vi "MotorMpas.vi"(2 "entrée d'erreur 2":errorcluster caption="entrée d'erreur", 3 "Parameter":i32) -> (0 "entrée d'erreur":errorcluster, 1 "Numérique":i32)   [LabVIEW 2009]
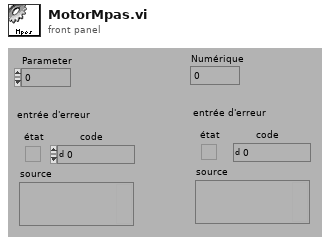
[diagram p1: front panel]
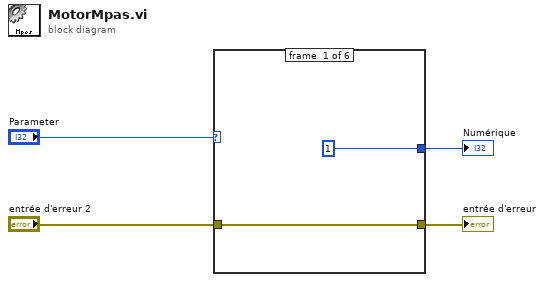
[diagram p0: block diagram]
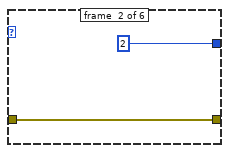
[diagram p2: hidden frame]
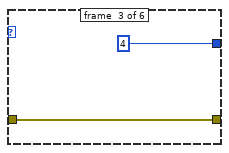
[diagram p3: hidden frame]
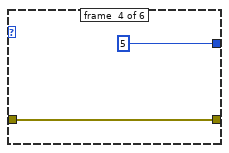
[diagram p4: hidden frame]
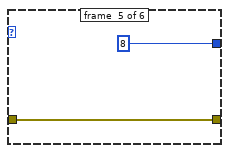
[diagram p5: hidden frame]
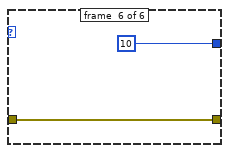
[diagram p6: hidden frame]
diagram:
  n1 = case shown="1, Default" "Parameter" {
    tunnel: "entrée d'erreur 2" -> [w6 w8 w10 w12 w14 w16]
    tunnel: [w6 w8 w10 w12 w14 w16] -> w4
    tunnel: [1 2 4 5 8 10] -> w3
    frame #0 {
    }
    frame #1 {
    }
    frame #2 {
    }
    frame #3 {
    }
    frame #4 {
    }
    frame #5 {
    }
  }
  "entrée d'erreur" <- w4
  "Numérique" <- w3
